vi "KE2260B Error Query.vi"(8 "error in (no error)":errorcluster, 11 "VISA resource name":refnum<visa-resource-name>) -> (0 "error out":errorcluster, 1 "Error Message":string, 2 "Error Code":i32[](array[numeric]), 3 "VISA resource name out":refnum<visa-resource-name>)   [LabVIEW 2021, in "Keithley 2260B.lvlib"]
doc: "Queries the instrument for any errors in the instrument's error queue. It will continue to read errors until all errors have been read from the instrument. Any errors will be returned in the <B>error out</B> control.\n\n<B>Note:</B>\nThis VI is called automatically by most driver VIs so it is not usually necessary to call this in an application."
uses:
  Keithley 2260B.lvlib
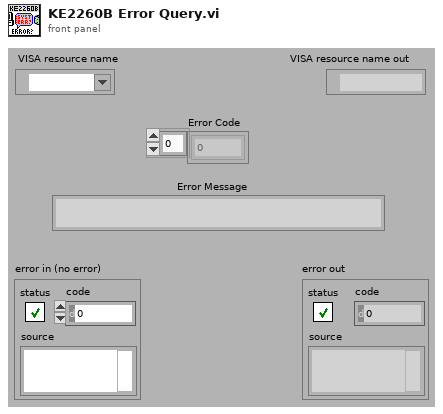
[diagram p1: front panel]
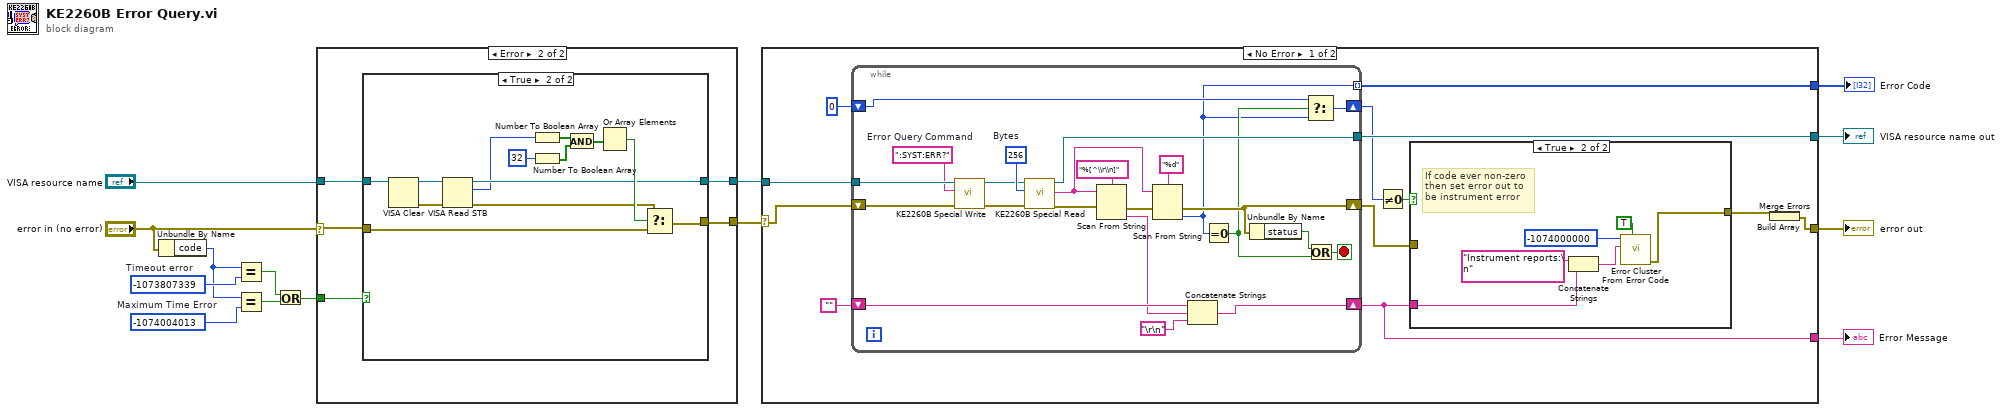
[diagram p0: block diagram]
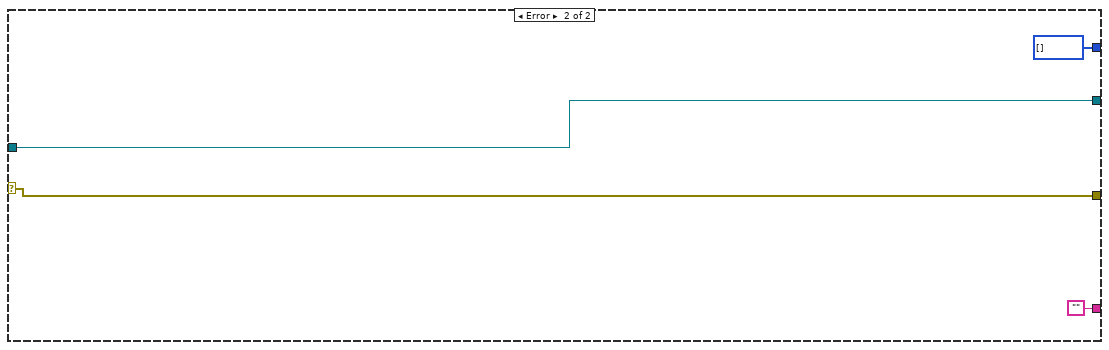
[diagram p5: hidden frame]
diagram:
  w5 = -1074004013  # Maximum Time Error
  w7 = -1073807339  # Timeout error
  n1 = Unbundle By Name("error in (no error)") -> ("code"=w6:i32)
  n2 = Equal?(x=w6, y=w7) -> (x = y?=w3:bool)
  n3 = Equal?(x=w6, y=w5) -> (x = y?=w4:bool)
  n4 = Or(x=w3, y=w4) -> (x .or. y?=w2:bool)
  n5 = case shown="Error" "error in (no error)" {
    selector: "error in (no error)" -> [w15 w19]
    tunnel: "VISA resource name" -> [w16 w21]
    tunnel: [w16 w20] -> w9
    tunnel: [w15 w18] -> w10
    tunnel: w2 -> [_ w17]
    frame No Error {
    }
    frame Error {
      n6 = case shown="True" w17 {
        tunnel: w21 -> [w23 w29]
        tunnel: [w23 w26] -> w20
        tunnel: w19 -> [w22 w32]
        tunnel: [w22 w31] -> w18
        frame False {
          # "Error code not a timeout, so best to pass on to user."
        }
        frame True {
          n7 = VISA Clear(VISA resource name=w29) -> (VISA resource name out=w28:refnum<visa-resource-name>, error out=w27:errorcluster)  [unwired: 1 in]
          n8 = VISA Read STB(8:w27, 11:w28) -> (0:w25:errorcluster, 2:w24:u16, 3:w26:refnum<visa-resource-name>)
          n9 = Number To Boolean Array(number=w24) -> (Boolean array=w33:bool[])
          n10 = Number To Boolean Array(number=32) -> (Boolean array=w35:bool[])
          n11 = And(x=w33, y=w35) -> (x .and. y?=w34:bool[])
          n12 = Or Array Elements(Boolean array=w34) -> (logical OR=w30:bool)
          n13 = Select(t=w25, s=w30, f=w32) -> (s? t:f=w31:errorcluster)
        }
      }
    }
  }
  n14 = case shown="No Error" w10 {
    selector: w10 -> [w38 w80]
    tunnel: [w49 w83] -> w14
    tunnel: w9 -> [w48 w83]
    tunnel: [w46 w80] -> w13
    tunnel: [w41 ""] -> w12
    tunnel: [w40 i32[] []] -> w11
    frame No Error {
      n15 = while {
        tunnel: [w79] -> w49
        tunnel: w48 -> [w59]
        shift-right: [w70] -> w41
        shift-left: "" -> [w73]
        shift-right: [w68] -> w42
        shift-left: 0 -> [w69]
        shift-right: [w67] -> w39
        shift-left: w38 -> [w58]
        tunnel: [w62] -> w40 mode=indexing
        stop <- w76 stop-if-true
        w78 = u32 256  # Bytes
        w57 = ":SYST:ERR?"  # Error Query Command
        n16 = call "KE2260B Special Write.vi"("error in (no error)"=w58, "Write Buffer (\"\")"=w57, "VISA session"=w59) -> ("error out"=w60:errorcluster, "dup VISA session"=w61:refnum<visa-resource-name>)  [unwired: 6 in, 1 out]
        n17 = call "KE2260B Special Read.vi"("error in (no error)"=w60, "byte count"=w78, "VISA session"=w61) -> ("error out"=w66:errorcluster, "read buffer"=w74:string, "dup VISA session"=w79:refnum<visa-resource-name>)  [unwired: 5 in, 1 out]
        n18 = Scan From String(format string="%[^\\r\\n]", input string=w74, error in=w66) -> (error out=w65:errorcluster, output 1=w71:string)  [unwired: 2 in, 2 out]
        n19 = Scan From String(format string="%d", input string=w74, error in=w65) -> (error out=w67:errorcluster, output 1=w62:i32)  [unwired: 2 in, 2 out]
        n20 = Concatenate Strings(w73, w71, "\r\n") -> (w70:string)
        n21 = Equal To 0?(x=w62) -> (x = 0?=w63:bool)
        n22 = Unbundle By Name(w67) -> ("status"=w64:bool)
        n23 = Select(t=w69, s=w63, f=w62) -> (s? t:f=w68:i32)
        n24 = Or(x=w64, y=w63) -> (x .or. y?=w76:bool)
      }
      n25 = Not Equal To 0?(x=w42) -> (x != 0?=w44:bool)
      n26 = case shown="True" w44 {
        tunnel: w41 -> [_ w55]
        tunnel: [w50 w51] -> w43
        tunnel: w39 -> [w50 _]
        frame False {
        }
        frame True {
          # "If code ever non-zero\nthen set error out to\nbe instrument error"
          n27 = Concatenate Strings("Instrument reports:\n" ("Source"), w55) -> (w52:string)
          n28 = call <vilib>:"Error Cluster From Error Code.vi"("show call chain? (False)"=TRUE, "error message (\"\")"=w52, "error code (0)"=-1074000000 ("Code")) -> ("error out"=w51:errorcluster)  [unwired: 6 in]
        }
      }
      n29 = Build Array(w43) -> (w37:errorcluster[])
      n30 = Merge Errors(w37) -> (w46:errorcluster)
    }
    frame Error {
    }
  }
  "VISA resource name out" <- w14
  "error out" <- w13
  "Error Message" <- w12
  "Error Code" <- w11
